vi "CalGas Auswahl - Strings zuweisen.vi"(7 "NUR Aufschaltung CalGas":bool, 9 "Def.CalGas":T1 {"Messbereiche"."Messbereich 12" items=["0-100ppm", "0-1000ppm", "0-5000ppm"]; "Messbereiche"."Messbereich 11" items=["0-100ppm", "0-1000ppm", "0-5000ppm"]; "Messbereiche"."Messbereich 10" items=["0-100ppm", "0-1000ppm", "0-5000ppm"]; "Messbereiche"."Messbereich 9" items=["0-100ppm", "0-1000ppm", "0-5000ppm"]; "Messbereiche"."Messbereich 8" items=["0-100ppm", "0-1000ppm", "0-5000ppm"]; "Messbereiche"."Messbereich 7" items=["0-100ppm", "0-1000ppm", "0-5000ppm"]; "Messbereiche"."Messbereich 6" items=["0-100ppm", "0-1000ppm", "0-5000ppm"]; "Messbereiche"."Messbereich 5" items=["0-100ppm", "0-1000ppm", "0-5000ppm"]; "Messbereiche"."Messbereich 4" items=["0-100ppm", "0-1000ppm", "0-5000ppm"]; "Messbereiche"."Messbereich 3" items=["0-100ppm", "0-1000ppm", "0-5000ppm"]; "Messbereiche"."Messbereich 2" items=["0-100ppm", "0-1000ppm", "0-5000ppm"]; "Messbereiche"."Messbereich 1" items=["0-100ppm", "0-1000ppm", "0-5000ppm"]; "Einheit"."Einheit 12" items=["ppm", "%"]; "Einheit"."Einheit 11" items=["ppm", "%"]; "Einheit"."Einheit 10" items=["ppm", "%"]; "Einheit"."Einheit 9" items=["ppm", "%"]; "Einheit"."Einheit 8" items=["ppm", "%"]; "Einheit"."Einheit 7" items=["ppm", "%"]; "Einheit"."Einheit 6" items=["ppm", "%"]; "Einheit"."Einheit 5" items=["ppm", "%"]; "Einheit"."Einheit 4" items=["ppm", "%"]; "Einheit"."Einheit 3" items=["ppm", "%"]; "Einheit"."Einheit 2" items=["ppm", "%"]; "Einheit"."Einheit 1" items=["ppm", "%"]; "Werte 2"."Konzentration 12" format="%#_5g"; "Werte 2"."Konzentration 11" format="%#_5g"; "Werte 2"."Konzentration 10" format="%#_5g"; "Werte 2"."Konzentration 9" format="%#_5g"; "Werte 2"."Konzentration 8" format="%#_5g"; "Werte 2"."Konzentration 7" format="%#_5g"; "Werte 2"."Konzentration 6" format="%#_5g"; "Werte 2"."Konzentration 5" format="%#_5g"; "Werte 2"."Konzentration 4" format="%#_5g"; "Werte 2"."Konzentration 3" format="%#_5g"; "Werte 2"."Konzentration 2" format="%#_5g"; "Werte 2"."Konzentration 1" format="%#_5g"; "Werte"."Konzentration 12" format="%#_5g"; "Werte"."Konzentration 11" format="%#_5g"; "Werte"."Konzentration 10" format="%#_5g"; "Werte"."Konzentration 9" format="%#_5g"; "Werte"."Konzentration 8" format="%#_5g"; "Werte"."Konzentration 7" format="%#_5g"; "Werte"."Konzentration 6" format="%#_5g"; "Werte"."Konzentration 5" format="%#_5g"; "Werte"."Konzentration 4" format="%#_5g"; "Werte"."Konzentration 3" format="%#_5g"; "Werte"."Konzentration 2" format="%#_5g"; "Werte"."Konzentration 1" format="%#_5g"}, 10 "Def.CalGas":refnum<vi>[](array[refnum]), 11 "Aufschaltung CalGas":refnum<vi>[](array[refnum])) -> (0 "Fehler (Ausgang)":errorcluster)   [LabVIEW 2020, in "CalGas Aufschaltung.lvlib"]
uses:
  CalGas Aufschaltung.lvlib
  Definition CalGas Anzeige.ctl
  CalGas-Namen.ctl
  Visualisierungs Elemente/String - Eingabefeld.ctl
  CalGas-Werte.ctl
  Visualisierungs Elemente/Zahlen-Eingabefeld.ctl
  CalGas-Einheit.ctl
  Visualisierungs Elemente/Auswahlfeld.ctl
  CalGas-Messbereiche.ctl
  Analysator Definition/FGV Analysator Definition Aktionen.ctl
  Sprachverwaltung/FGV Aktion Tabelle zerlegen.ctl
  FGV CalGas Aktionen.ctl
  Analysator Definition/Analysator Definition.lvlib
  Sprachverwaltung/Sprachverwaltung.lvlib
panel:
  out "Strings [] 5":string[][](array[string])
  # "Span 1"
  # "Span 2"
  # "Span 3"
  # "Span 4"
  # "Span 5"
  # "Span 6"
  # "Span 7"
  # "Span 8"
  # "Span 9"
  # "Span 10"
  # "Span 11"
  # "Span 12"
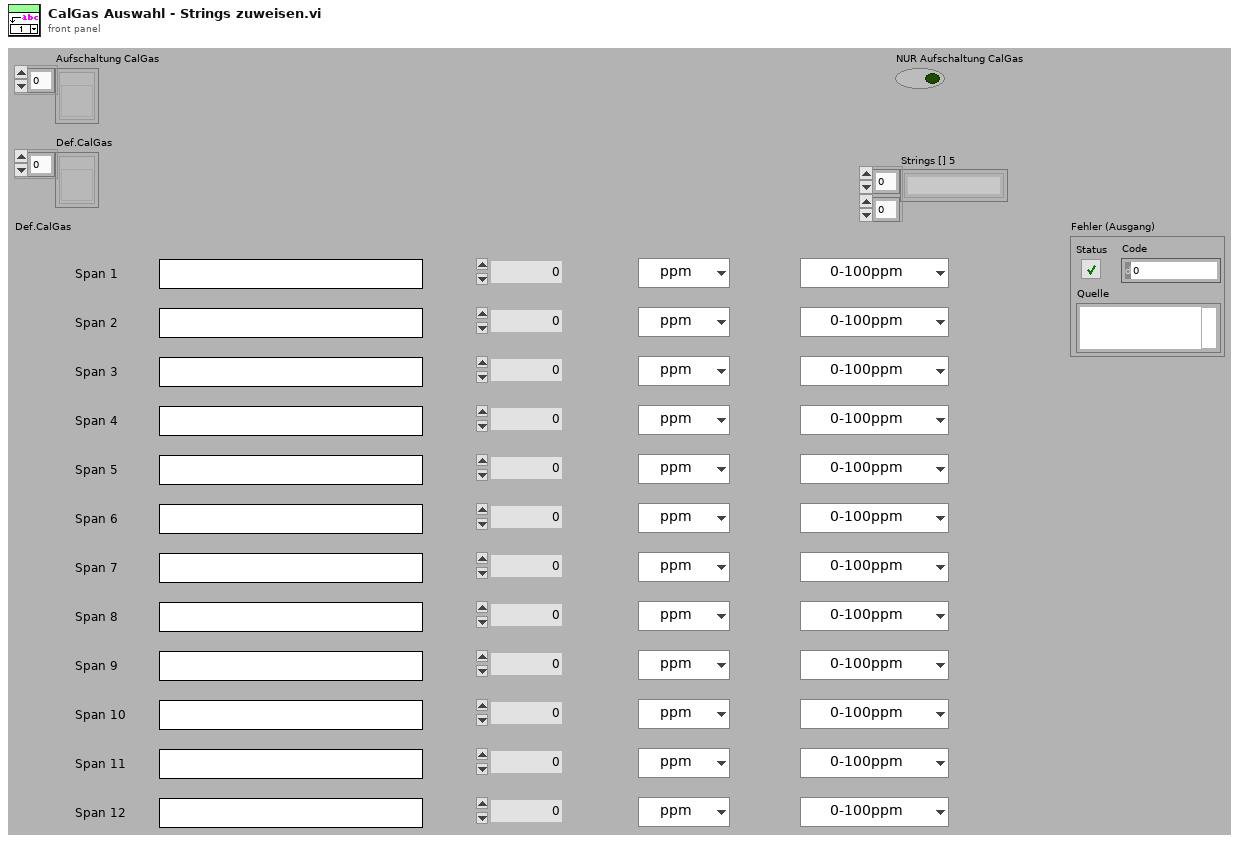
[diagram p1: front panel]
types:
  T1 = typedef "CalGas Aufschaltung.lvlib/Definition CalGas Anzeige.ctl" = cluster{"Namen":T2, "Werte":T4, "Werte 2":T4, "Einheit":T6, "Messbereiche":T8}
  T2 = typedef "CalGas Aufschaltung.lvlib/CalGas-Namen.ctl" = cluster{"Name":T3, "Name 2":T3, "Name 3":T3, "Name 4":T3, "Name 5":T3, "Name 6":T3, "Name 7":T3, "Name 8":T3, "Name 9":T3, "Name 10":T3, "Name 11":T3, "Name 12":T3}
  T3 = typedef "String - Eingabefeld.ctl" = string
  T4 = typedef "CalGas Aufschaltung.lvlib/CalGas-Werte.ctl" = cluster{"Konzentration 1":T5, "Konzentration 2":T5, "Konzentration 3":T5, "Konzentration 4":T5, "Konzentration 5":T5, "Konzentration 6":T5, "Konzentration 7":T5, "Konzentration 8":T5, "Konzentration 9":T5, "Konzentration 10":T5, "Konzentration 11":T5, "Konzentration 12":T5}
  T5 = typedef "Zahlen-Eingabefeld.ctl" = sgl
  T6 = typedef "CalGas Aufschaltung.lvlib/CalGas-Einheit.ctl" = cluster{"Einheit 1":T7, "Einheit 2":T7, "Einheit 3":T7, "Einheit 4":T7, "Einheit 5":T7, "Einheit 6":T7, "Einheit 7":T7, "Einheit 8":T7, "Einheit 9":T7, "Einheit 10":T7, "Einheit 11":T7, "Einheit 12":T7}
  T7 = typedef "Auswahlfeld.ctl" = u16
  T8 = typedef "CalGas Aufschaltung.lvlib/CalGas-Messbereiche.ctl" = cluster{"Messbereich 1":T7, "Messbereich 2":T7, "Messbereich 3":T7, "Messbereich 4":T7, "Messbereich 5":T7, "Messbereich 6":T7, "Messbereich 7":T7, "Messbereich 8":T7, "Messbereich 9":T7, "Messbereich 10":T7, "Messbereich 11":T7, "Messbereich 12":T7}
  T9 = typedef "Sprachverwaltung.lvlib/FGV Aktion Tabelle zerlegen.ctl" = enum16{"laden", "vereinzeln", "speichern"}
  T10 = typedef "Analysator Definition.lvlib/FGV Analysator Definition Aktionen.ctl" = enum16{"lesen", "MB setzen", "MB KAL setzen", "laden"}
  T11 = typedef "Analysator Definition.lvlib/Betriebsdaten Komponente.ctl" = cluster{"Namen":string[], "MB Namen":string[], "Einheit":string, "MB Aktuell":u16, "MB Endwert":u16, "CalGase":u16[], "MB für KAL":u16[], "CG für KAL":u16[]}
  T12 = typedef "CalGas Aufschaltung.lvlib/FGV CalGas Aktionen.ctl" = enum16{"lesen", "Analysator Auswahl", "Def.CalGas", "Aufschaltung CalGas", "laden", "speichern", "KAL extrahieren"}
  T13 = enum8{"Enabled", "Disabled", "Disabled and Grayed Out"}
  T14 = typedef "CalGas Aufschaltung.lvlib/Cluster Auswahl Analysator.ctl" = cluster{"Analysator Auswahl":T15, "Analysator Auswahl 2":T15, "Analysator Auswahl 3":T15, "Analysator Auswahl 4":T15, "Analysator Auswahl 5":T15, "Analysator Auswahl 6":T15, "Analysator Auswahl 7":T15, "Analysator Auswahl 8":T15, "Analysator Auswahl 9":T15, "Analysator Auswahl 10":T15, "Analysator Auswahl 11":T15, "Analysator Auswahl 12":T15}
  T15 = typedef "CalGas Aufschaltung.lvlib/Analysator Auswahl.ctl" = u16
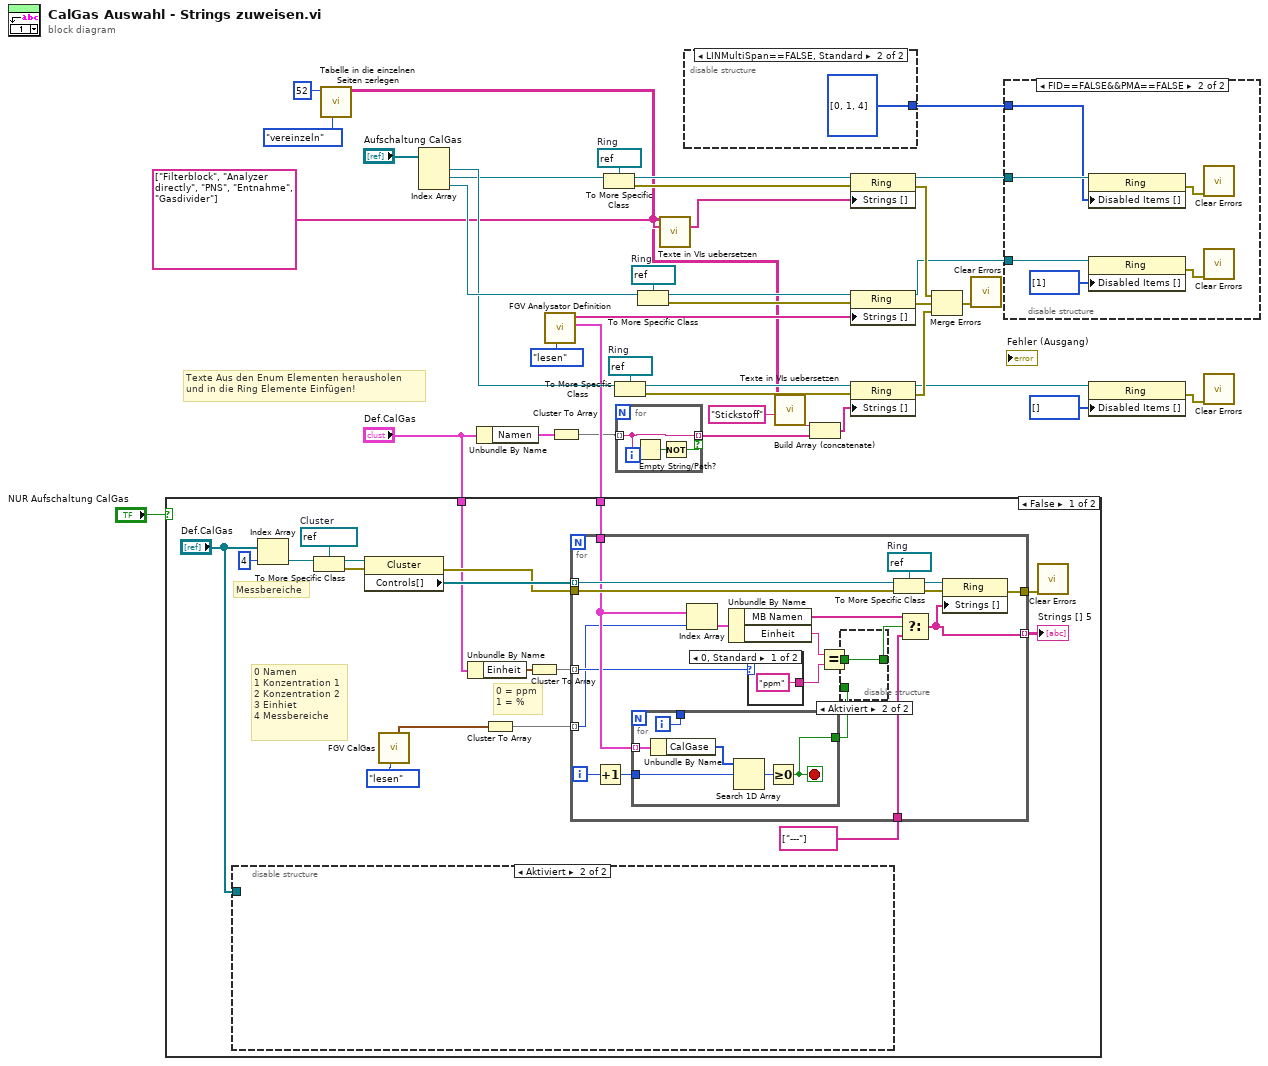
[diagram p0: block diagram]
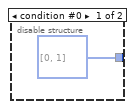
[diagram p2: hidden frame]
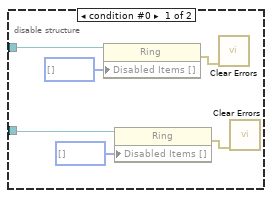
[diagram p3: hidden frame]
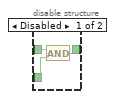
[diagram p4: hidden frame]
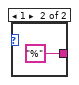
[diagram p5: hidden frame]
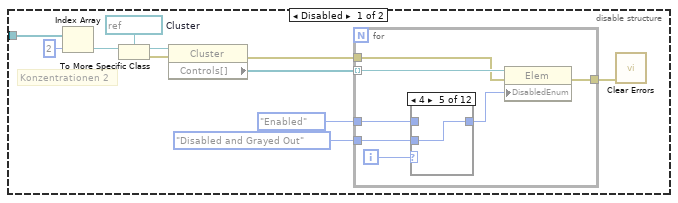
[diagram p6: hidden frame]
diagram:
  w34 = refnum<vi> refnum  # Ring
  w35 = refnum<vi> refnum  # Ring
  w39 = refnum<vi> refnum  # Ring
  # "Texte Aus den Enum Elementen herausholen \nund in die Ring Elemente Einfügen!"
  n1 = call "Tabelle in die einzelnen Seiten zerlegen.vi"("Aktion"=FGV_Aktion_Tabelle_zerlegen."vereinzeln", "Index (Seite)"=52) -> ("Sprachliste"=w11:string[][])  [unwired: 7 in, 2 out]
  n2 = Index Array(array="Aufschaltung CalGas") -> (element #1=w20:refnum<vi>, element #2=w19:refnum<vi>, element #3=w32:refnum<vi>)  [unwired: 3 in]
  n3 = Unbundle By Name("Def.CalGas") -> ("Namen"=w30:T2)
  n4 = call "FGV Analysator Definition.vi"("Aktionen"=FGV_Analysator_Definition_Aktionen."lesen") -> ("Betriebsdaten"=w4:T11[], "Analysatoren"=w17:string[])  [unwired: 6 in, 3 out]
  n5 = case shown="False" "NUR Aufschaltung CalGas" {
    tunnel: "Def.CalGas" -> [w46 _]
    tunnel: w4 -> [w45 _]
    frame False {
      w56 = refnum<vi> refnum  # Cluster
      # "0 = ppm\n1 = %"
      # "0 Namen\n1 Konzentration 1\n2 Konzentration 2\n3 Einhiet\n4 Messbereiche"
      # "Messbereiche"
      n6 = disable-structure shown="Aktiviert" {
        disable-tunnel: "Def.CalGas" -> [w96 _]
        frame Disabled {
          w98 = refnum<vi> refnum  # Cluster
          # "Konzentrationen 2"
          n7 = Index Array(array=w96, index=2 ("Index")) -> (element=w100:refnum<vi>)
          n8 = To More Specific Class(target class=w98, reference=w100) -> (specific class reference=w99:refnum<vi>, error out=w92:errorcluster)  [unwired: 1 in]
          n9 = property class="Cluster"(reference=w99, error in=w92) -> (error out=w90:errorcluster, "Controls[]"=w95:refnum<vi>[])  [unwired: 1 out]
          n10 = for {
            tunnel: w95 -> [w107] mode=indexing
            tunnel: T13."Disabled and Grayed Out" ("Deaktiviert") -> [w105]
            tunnel: T13."Enabled" ("Deaktiviert") -> [w104]
            tunnel: [w102] -> w91
            tunnel: w90 -> [w101]
            i -> [w106]
            n11 = case shown="4" w106 {
              tunnel: w105 -> [_ _ _ _ w112 w113 w114 w115 w116 w117 w118 w119]
              tunnel: w104 -> [w108 w109 w110 w111 _ _ _ _ _ _ _ _]
              tunnel: [w108 w109 w110 w111 w112 w113 w114 w115 w116 w117 w118 w119] -> w103
              frame 0, Default {
              }
              frame 1 {
              }
              frame 2 {
              }
              frame 3 {
              }
              frame 4 {
              }
              frame 5 {
              }
              frame 6 {
              }
              frame 7 {
              }
              frame 8 {
              }
              frame 10 {
              }
              frame 11 {
              }
              frame 9 {
              }
            }
            n12 = property class="Elem"(reference=w107, error in=w101, "DisabledEnum"=w103) -> (error out=w102:errorcluster)  [unwired: 1 out]
          }
          n13 = call <vilib>:"Clear Errors.vi"("error in (no error)"=w91) -> ()  [unwired: 5 in, 2 out]
        }
        frame Enabled {
        }
      }
      n14 = Index Array(array="Def.CalGas", index=4 ("Index")) -> (element=w55:refnum<vi>)
      n15 = To More Specific Class(target class=w56, reference=w55) -> (specific class reference=w47:refnum<vi>, error out=w44:errorcluster)  [unwired: 1 in]
      n16 = property class="Cluster"(reference=w47, error in=w44) -> (error out=w48:errorcluster, "Controls[]"=w52:refnum<vi>[])  [unwired: 1 out]
      n17 = call "FGV CalGas.vi"("Aktionen"=FGV_CalGas_Aktionen."lesen") -> ("Analysator Auswahl"=w42:T14)  [unwired: 6 in, 4 out]
      n18 = Unbundle By Name(w46) -> ("Einheit"=w51:T6)
      n19 = Cluster To Array(cluster=w42) -> (array=w41:T15[])
      n20 = Cluster To Array(cluster=w51) -> (array=w50:T7[])
      n21 = for {
        tunnel: w52 -> [w75] mode=indexing
        tunnel: w50 -> [w63] mode=indexing
        tunnel: [w73] -> w49
        tunnel: w48 -> [w72]
        tunnel: string[] ["---"] ("Strings [] 5") -> [w67]
        tunnel: w45 -> [w64]
        tunnel: w41 -> [w59] mode=indexing
        tunnel: [w58] -> w40 mode=indexing
        i -> [w71]
        w77 = refnum<vi> refnum  # Ring
        n22 = Increment(x=w71) -> (x+1=w70:i32)
        n23 = for {
          tunnel: w64 -> [w89] mode=indexing
          tunnel: w70 -> [w87]
          tunnel: [w85] -> _
          tunnel: [w84] -> w66
          i -> [w85]
          stop <- w84 stop-if-true
          n24 = Unbundle By Name(w89) -> ("CalGase"=w88:u16[])
          n25 = Search 1D Array(1D array=w88, element=w87) -> (index of element=w86:i32)  [unwired: 1 in]
          n26 = Greater Or Equal To 0?(x=w86) -> (x >= 0?=w84:bool)
        }
        n27 = Index Array(array=w64, index=w59) -> (element=w69:T11)
        n28 = Unbundle By Name(w69) -> ("MB Namen"=w68:string[], "Einheit"=w62:string)
        n29 = case shown="0, Standard" w63 {
          tunnel: ["ppm" "%"] -> w60
          frame 0, Default {
          }
          frame 1 {
          }
        }
        n30 = Equal?(x=w62, y=w60) -> (x = y?=w61:bool)
        n31 = disable-structure shown="Aktiviert" {
          disable-tunnel: w66 -> [w80 _]
          disable-tunnel: [w79 w81] -> w65
          disable-tunnel: w61 -> [w78 w81]
          frame Disabled {
            n32 = And(x=w78, y=w80) -> (x .and. y?=w79:bool)
          }
          frame Enabled {
          }
        }
        n33 = To More Specific Class(target class=w77, reference=w75, error in=w72) -> (specific class reference=w76:refnum<vi>, error out=w74:errorcluster)
        n34 = Select(t=w68, s=w65, f=w67) -> (s? t:f=w58:string[])
        n35 = property class="Ring"(reference=w76, error in=w74, "Strings []"=w58) -> (error out=w73:errorcluster)  [unwired: 1 out]
      }
      "Strings [] 5" <- w40
      n36 = call <vilib>:"Clear Errors.vi"("error in (no error)"=w49) -> ()  [unwired: 5 in, 2 out]
    }
    frame True {
    }
  }
  n37 = Cluster To Array(cluster=w30) -> (array=w3:T3[])
  n38 = To More Specific Class(target class=w34, reference=w19) -> (specific class reference=w33:refnum<vi>, error out=w29:errorcluster)  [unwired: 1 in]
  n39 = To More Specific Class(target class=w39, reference=w20) -> (specific class reference=w38:refnum<vi>, error out=w27:errorcluster)  [unwired: 1 in]
  n40 = for {
    tunnel: w3 -> [w122] mode=indexing
    tunnel: [w122] -> w2 mode=indexing if=w120
    n41 = Empty String/Path?(string/path=w122) -> (empty?=w121:bool)
    n42 = Not(x=w121) -> (.not. x?=w120:bool)
  }
  n43 = To More Specific Class(target class=w35, reference=w32) -> (specific class reference=w36:refnum<vi>, error out=w28:errorcluster)  [unwired: 1 in]
  n44 = call "Texte in VIs uebersetzen.vi"("Sprachliste"=w11, "String-Array zum Übersetzen"=string[] ["Filterblock", "Analyzer directly", "PNS", "Entnahme", "Gasdivider"] ("Strings []")) -> ("String-Array zum Übersetzen"=w14:string[])  [unwired: 9 in, 4 out]
  n45 = disable-structure shown="LINMultiSpan==FALSE, Standard" {
    disable-tunnel: [i32[] [0, 1] ("Deaktivierte Objekte []") i32[] [0, 1, 4] ("Deaktivierte Objekte []")] -> w1
    frame condition #0 {
    }
    frame condition #1 (active) {
    }
  }
  n46 = call "Texte in VIs uebersetzen.vi"("Sprachliste"=w11, "String zum Übersetzen"="Stickstoff" ("String")) -> ("String zum Übersetzen"=w12:string)  [unwired: 9 in, 4 out]
  n47 = Build Array (concatenate)(w12, w2) -> (w31:T3[])
  n48 = property class="Ring"(reference=w33, error in=w29, "Strings []"=w14) -> (reference out=w9:refnum<vi>, error out=w26:errorcluster)
  n49 = property class="Ring"(reference=w36, error in=w28, "Strings []"=w17) -> (reference out=w5:refnum<vi>, error out=w25:errorcluster)
  n50 = property class="Ring"(reference=w38, error in=w27, "Strings []"=w31) -> (reference out=w7:refnum<vi>, error out=w24:errorcluster)
  n51 = Merge Errors(w26, w25, w24) -> (w23:errorcluster)
  n52 = call <vilib>:"Clear Errors.vi"("error in (no error)"=w23) -> ()  [unwired: 5 in, 2 out]
  n53 = disable-structure shown="FID==FALSE&&PMA==FALSE" {
    disable-tunnel: w9 -> [w129 w136]
    disable-tunnel: w5 -> [w125 w132]
    disable-tunnel: w1 -> [_ w131]
    frame condition #0 {
      n54 = property on="Eigenschaftsknoten" class="Ring"(reference=w129, "Disabled Items []"=i32[] [] ("Deaktivierte Objekte []")) -> (error out=w130:errorcluster)  [unwired: 1 in, 1 out]
      n55 = property on="Eigenschaftsknoten" class="Ring"(reference=w125, "Disabled Items []"=i32[] [] ("Deaktivierte Objekte []")) -> (error out=w126:errorcluster)  [unwired: 1 in, 1 out]
      n56 = call <vilib>:"Clear Errors.vi"("error in (no error)"=w130) -> ()  [unwired: 5 in, 2 out]
      n57 = call <vilib>:"Clear Errors.vi"("error in (no error)"=w126) -> ()  [unwired: 5 in, 2 out]
    }
    frame condition #1 (active) {
      n58 = property on="Eigenschaftsknoten" class="Ring"(reference=w136, "Disabled Items []"=w131) -> (error out=w135:errorcluster)  [unwired: 1 in, 1 out]
      n59 = property on="Eigenschaftsknoten" class="Ring"(reference=w132, "Disabled Items []"=i32[] [1] ("Deaktivierte Objekte []")) -> (error out=w134:errorcluster)  [unwired: 1 in, 1 out]
      n60 = call <vilib>:"Clear Errors.vi"("error in (no error)"=w135) -> ()  [unwired: 5 in, 2 out]
      n61 = call <vilib>:"Clear Errors.vi"("error in (no error)"=w134) -> ()  [unwired: 5 in, 2 out]
    }
  }
  n62 = property on="Eigenschaftsknoten" class="Ring"(reference=w7, "Disabled Items []"=i32[] [] ("Deaktivierte Objekte []")) -> (error out=w8:errorcluster)  [unwired: 1 in, 1 out]
  n63 = call <vilib>:"Clear Errors.vi"("error in (no error)"=w8) -> ()  [unwired: 5 in, 2 out]
